vi "Type Conversion.From Double (1D U16).vi"(3 "values in":dbl[](array[numeric])) -> (1 "values out":u16[](array[numeric]))   [LabVIEW 2016, in "VeriStand Data.lvlib"]
doc: "Converts the provided double float values to the specified data type, preserving the numerical value of the data."
uses:
  VeriStand Data.lvlib
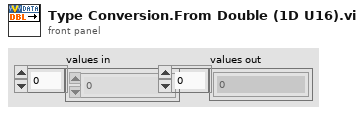
[diagram p1: front panel]
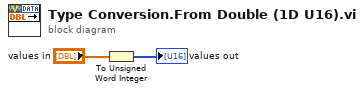
[diagram p0: block diagram]
diagram:
  n1 = To Unsigned Word Integer(number="values in") -> (unsigned 16bit integer=→"values out":u16[])
